vi "Acquire Data.vi"(7 "Total Buffer Size":i32 caption="全部缓冲区大小", 8 "error in (no error)":errorcluster caption="错误输入（无错误）", 10 "Acquisition and Logging Configuration":T2={"Samples per Read"=100, "Number of Reads to Save"=20, "Number of Channels"=4, "Channel Scale Array"=[1.0, 1.0, 1.0, 1.0], "Channel Names"=["Mod1\\AI0", "Mod1\\AI1", "Mod1\\AI2", "Mod1\\AI3"], "Trigger - RMS Value"=0.9999999999999994, "Trigger - Channel"=0, "Trigger - Time (Minute)"=10, "TDMS Properties"=[{"Name"="Company", "Value"="TongRui"}, {"Name"="Developer", "Value"="SUN"}], "Data File Name"="cRIO_Data", "Date Rate"=20} caption="采集与记录配置" {"Date Rate" items=["51.200 kS/s (NI 9234)"=1, "25.600 kS/s (NI 9234)"=2, "17.067 kS/s (NI 9234)"=3, "12.80 kS/s (NI 9234)"=4, "10.240 kS/s (NI 9234)"=5, "8.533 kS/s (NI 9234)"=6, "7.314 kS/s (NI 9234)"=7, "6.400 kS/s (NI 9234)"=8, "5.689 kS/s (NI 9234)"=9, "5.120 kS/s (NI 9234)"=10, "4.654 kS/s (NI 9234)"=11, "4.267 kS/s (NI 9234)"=12, "3.938 kS/s (NI 9234)"=13, "3.657 kS/s (NI 9234)"=14, "3.413 kS/s (NI 9234)"=15, "3.200 kS/s (NI 9234)"=16, "3.012 kS/s (NI 9234)"=17, "2.845 kS/s (NI 9234)"=18, "2.695 kS/s (NI 9234)"=19, "2.560 kS/s (NI 9234)"=20, "2.438 kS/s (NI 9234)"=21, "2.328 kS/s (NI 9234)"=22, "2.226 kS/s (NI 9234)"=23, "2.133 kS/s (NI 9234)"=24, "2.048 kS/s (NI 9234)"=25, "1.969 kS/s (NI 9234)"=26, "1.896 kS/s (NI 9234)"=27, "1.829 kS/s (NI 9234)"=28, "1.765 kS/s (NI 9234)"=29, "1.707 kS/s (NI 9234)"=30, "1.652 kS/s (NI 9234)"=31]}, 11 "FPGA VI Reference":T1 caption="FPGA VI引用") -> (0 "error out":errorcluster caption="错误输出", 1 "Waveform Data":waveform(sgl)[](array[waveform]) caption="波形数据", 2 "dup Acquisition and Logging Configuration":T2={"Samples per Read"=100, "Number of Reads to Save"=20, "Number of Channels"=4, "Channel Scale Array"=[1.0, 1.0, 1.0, 1.0], "Channel Names"=[], "Trigger - RMS Value"=0.9999999999999994, "Trigger - Channel"=0, "Trigger - Time (Minute)"=10, "TDMS Properties"=[], "Data File Name"="cRIO_Data", "Date Rate"=20} caption="采集与记录配置副本" {"Date Rate" items=["51.200 kS/s (NI 9234)"=1, "25.600 kS/s (NI 9234)"=2, "17.067 kS/s (NI 9234)"=3, "12.80 kS/s (NI 9234)"=4, "10.240 kS/s (NI 9234)"=5, "8.533 kS/s (NI 9234)"=6, "7.314 kS/s (NI 9234)"=7, "6.400 kS/s (NI 9234)"=8, "5.689 kS/s (NI 9234)"=9, "5.120 kS/s (NI 9234)"=10, "4.654 kS/s (NI 9234)"=11, "4.267 kS/s (NI 9234)"=12, "3.938 kS/s (NI 9234)"=13, "3.657 kS/s (NI 9234)"=14, "3.413 kS/s (NI 9234)"=15, "3.200 kS/s (NI 9234)"=16, "3.012 kS/s (NI 9234)"=17, "2.845 kS/s (NI 9234)"=18, "2.695 kS/s (NI 9234)"=19, "2.560 kS/s (NI 9234)"=20, "2.438 kS/s (NI 9234)"=21, "2.328 kS/s (NI 9234)"=22, "2.226 kS/s (NI 9234)"=23, "2.133 kS/s (NI 9234)"=24, "2.048 kS/s (NI 9234)"=25, "1.969 kS/s (NI 9234)"=26, "1.896 kS/s (NI 9234)"=27, "1.829 kS/s (NI 9234)"=28, "1.765 kS/s (NI 9234)"=29, "1.707 kS/s (NI 9234)"=30, "1.652 kS/s (NI 9234)"=31]})   [LabVIEW 2013]
doc: "读取DMA FIFO的波形数据。"
uses:
  controls/Acquisition and Logging Configuration.ctl
  controls/TDMS Properties.ctl
  <vilib>/LabVIEW Targets/FPGA/cRIO/shared/nicrio_ModuleControls/nicrio_cRIO-9234_DataRatesRing2.ctl
  controls/FPGA VI Reference.ctl
  <vilib>/rvi/interface/common/niFpgaWaitOnOcc.vi
  Globals/Global - Monitoring Variables.vi
  <vilib>/Utility/error.llb/Error Cluster From Error Code.vi
  <vilib>/rvi/errors/niLvFpgaAdjustHostInterfaceError.vi
  <vilib>/rvi/interface/nirviReadWriteControl/nirviReadWriteControl.xnode
  FPGA Bitfiles/LabVIEWFPGAWavef_FPGA_FPGAMain_vTbN89OLNVY.lvbitx
  FPGA Main.vi
  <vilib>/rvi/interface/nirviMethod/nirviMethod.xnode
  NiFpgaLv.dll
  <vilib>/FPGAPlugInAG/cRIO-9074/niLvFpga_ReadFifo_cRIO-9074.vi
  <vilib>/rvi/errors/niLvFpgaMergeErrorWithErrorCode.vi
panel:
  # "通道"
  # "保存"
  # "采样"
  # "触发"
  # "通道"
  # "保存"
  # "采样"
  # "触发"
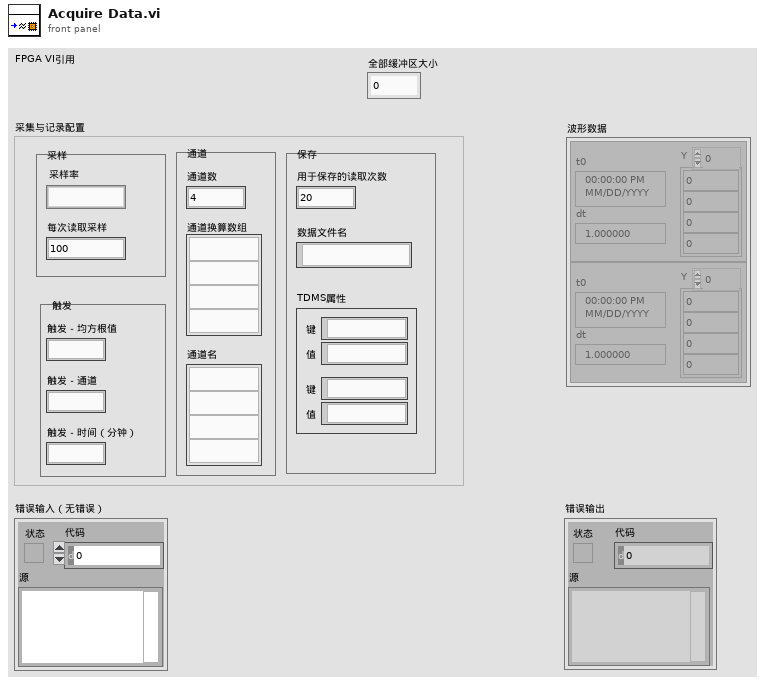
[diagram p1: front panel]
types:
  T1 = typedef "FPGA VI Reference.ctl" = refnum<k20>
  T2 = typedef "Acquisition and Logging Configuration.ctl" = cluster{"Samples per Read":i32, "Number of Reads to Save":i32, "Number of Channels":i32, "Channel Scale Array":fxp<+,24,12>[], "Channel Names":string[], "Trigger - RMS Value":dbl, "Trigger - Channel":i32, "Trigger - Time (Minute)":i32, "TDMS Properties":T3[], "Data File Name":string, "Date Rate":T4}
  T3 = typedef "TDMS Properties.ctl" = cluster{"Name":string, "Value":string}
  T4 = typedef "nicrio_cRIO-9234_DataRatesRing2.ctl" = u16
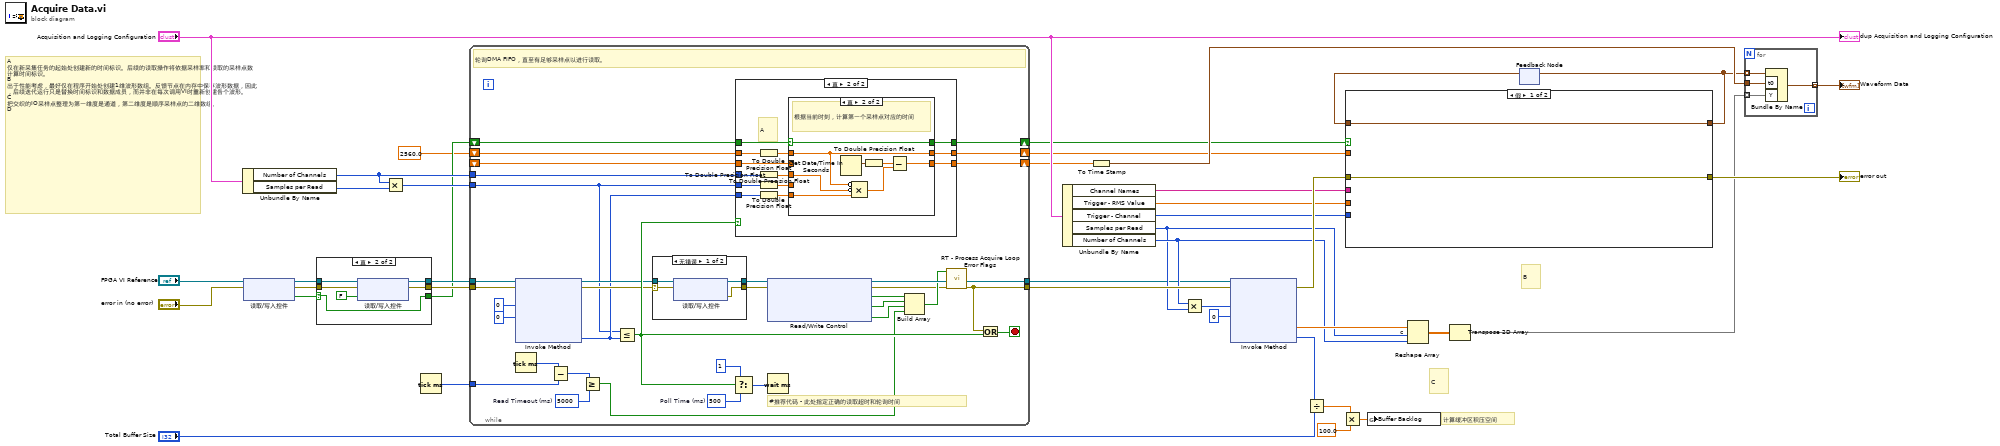
[diagram p0: block diagram]
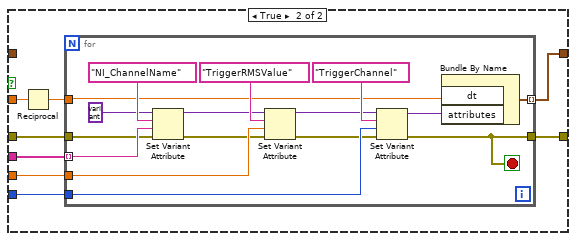
[diagram p2: hidden frame]
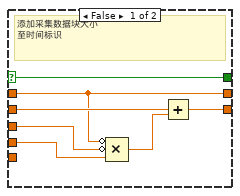
[diagram p5: hidden frame]
diagram:
  # "C"
  # "B"
  # "A\n仅在新采集任务的起始处创建新的时间标识。后续的读取操作将依据采样率和读取的采样点数计算时间标识。\nB\n出于性能考虑，最好仅在程序开始处创建1维波形数组。反馈节点在内存中保存波形数据，因此，后续迭代运行只是替换时间标识和数据成员，而并非在每次调用VI时重新创建各个波形。\nC\n把交织的IO采样点整理为第一维度是通道，第二维度是顺序采样点的二维数组。\nD"
  # "计算缓冲区积压空间"
  # "c"
  n1 = Unbundle By Name("Acquisition and Logging Configuration") -> ("Number of Channels"=w14:i32, "Samples per Read"=w15:i32)
  n2 = xnode "读取/写入控件"("FPGA VI引用输入"="FPGA VI Reference", "错误输入"="error in (no error)") -> ("FPGA VI引用输出"=w38:T1, "错误输出"=w39:errorcluster, "First Read"=w11:bool)
  n3 = case shown="真" w11 {
    selector: w11 -> [w41 w45]
    tunnel: w38 -> [w43 w49]
    tunnel: [w43 w48] -> w36
    tunnel: w39 -> [w42 w47]
    tunnel: [w42 w46] -> w35
    tunnel: [w41 w45] -> w10
    frame False {
    }
    frame True {
      n4 = xnode "读取/写入控件"("FPGA VI引用输入"=w49, "错误输入"=w47, "First Read"=FALSE) -> ("FPGA VI引用输出"=w48:T1, "错误输出"=w46:errorcluster)
    }
  }
  n5 = Multiply(x=w14, y=w15) -> (x*y=w30:i32)
  n6 = Tick Count (ms)() -> (millisecond timer value=w34:u32)
  n7 = while {
    tunnel: [w61] -> w33
    tunnel: [w66] -> w1
    tunnel: w36 -> [w81]
    tunnel: w35 -> [w80]
    shift-right: [w74] -> w32
    shift-left: _ -> [w79]
    tunnel: w34 -> [w82]
    tunnel: w30 -> [w50]
    tunnel: w14 -> [w58]
    shift-right: [w54] -> w13
    shift-left: 2560.0 -> [w59]
    shift-right: [w52] -> w12
    shift-left: w10 -> [w53]
    stop <- w83 stop-if-true
    w55 = u32 5000  # Read Timeout (ms)
    w56 = u32 500  # Poll Time (ms)
    # "#推荐代码 - 此处指定正确的读取超时和轮询时间"
    # "轮询DMA FIFO，直至有足够采样点以进行读取。"
    n8 = xnode "Invoke Method"("FPGA VI引用输入"=w81, "错误输入"=w80, "元素数量"=u32 0 ("Number of Elements"), "超时(ms)"=0 ("Timeout (ms)")) -> ("FPGA VI引用输出"=w69:T1, "错误输出"=w70:errorcluster, "剩余元素"=w51:u32)  [unwired: 1 out]
    n9 = Tick Count (ms)() -> (millisecond timer value=w78:u32)
    n10 = Subtract(x=w78, y=w82) -> (x-y=w71:u32)
    n11 = Greater Or Equal?(x=w71, y=w55) -> (x >= y?=w57:bool)
    n12 = Less Or Equal?(x=w50, y=w51) -> (x <= y?=w77:bool)
    n13 = case shown="无错误" w70 {
      selector: w70 -> [w87 w88]
      tunnel: w69 -> [w86 w89]
      tunnel: [w85 w89] -> w68
      tunnel: [w84 w88] -> w67
      frame No Error {
        n14 = xnode "读取/写入控件"("FPGA VI引用输入"=w86, "错误输入"=w87) -> ("FPGA VI引用输出"=w85:T1, "FPGA Error"=w84:errorcluster)  [unwired: 1 out]
      }
      frame Error {
      }
    }
    n15 = Select(t=u32 1, s=w77, f=w56) -> (s? t:f=w76:u32)
    n16 = case shown="真" w77 {
      tunnel: w79 -> [w92 w105]
      tunnel: w53 -> [w90 w104]
      tunnel: w51 -> [_ w103]
      tunnel: [w92 w102] -> w74
      tunnel: w50 -> [_ w101]
      tunnel: w59 -> [w91 w99]
      tunnel: w58 -> [_ w98]
      tunnel: [w91 w95] -> w54
      tunnel: [w90 w94] -> w52
      frame False {
      }
      frame True {
        # "A"
        n17 = To Double Precision Float(number=w99) -> (double precision float=w93:dbl)
        n18 = To Double Precision Float(number=w98) -> (double precision float=w100:dbl)
        n19 = To Double Precision Float(number=w101) -> (double precision float=w96:dbl)
        n20 = To Double Precision Float(number=w103) -> (double precision float=w97:dbl)
        n21 = case shown="真" w104 {
          selector: w104 -> [w106 w113]
          tunnel: w93 -> [w108 w115]
          tunnel: w105 -> [w111 _]
          tunnel: w96 -> [w109 _]
          tunnel: w100 -> [w110 w120]
          tunnel: w97 -> [_ w116]
          tunnel: [w112 w118] -> w102
          tunnel: [w108 w115] -> w95
          tunnel: [w106 w113] -> w94
          frame False {
            # "添加采集数据块大小\n至时间标识"
            n22 = Compound Arithmetic op=MULTIPLY(invert w108, invert w110, w109) -> (w107:dbl)
            n23 = Add(x=w111, y=w107) -> (x+y=w112:dbl)
          }
          frame True {
            # "根据当前时刻，计算第一个采样点对应的时间"
            n24 = Get Date/Time In Seconds() -> (seconds since 1Jan1904=w119:timestamp)
            n25 = Compound Arithmetic op=MULTIPLY(invert w115, invert w120, w116) -> (w114:dbl)
            n26 = To Double Precision Float(number=w119) -> (double precision float=w117:dbl)
            n27 = Subtract(x=w117, y=w114) -> (x-y=w118:dbl)
          }
        }
      }
    }
    n28 = xnode "Read/Write Control"("FPGA VI引用输入"=w68, "错误输入"=w67) -> ("FPGA VI引用输出"=w66:T1, "错误输出"=w60:errorcluster, "Module Underflow"=w63:bool, "DMA FIFO Full"=w65:bool, "Different Channel Count"=w64:bool)
    n29 = Wait (ms)(milliseconds to wait=w76) -> ()  [unwired: 1 out]
    n30 = Build Array(w63, w65, w64, w57) -> (w62:bool[])
    n31 = call "RT - Process Acquire Loop Error Flags.vi"("error in (no error)"=w60, "Error Flags"=w62) -> ("error out"=w61:errorcluster)  [unwired: 9 in]
    n32 = Or(x=w61, y=w77) -> (x .or. y?=w83:bool)
  }
  n33 = Unbundle By Name("Acquisition and Logging Configuration") -> ("Channel Names"=w4:string[], "Trigger - RMS Value"=w5:dbl, "Trigger - Channel"=w6:i32, "Samples per Read"=w7:i32, "Number of Channels"=w8:i32)
  n34 = To Time Stamp(1:w32) -> (0:w24:timestamp)
  n35 = Multiply(x=w8, y=w7) -> (x*y=w9:i32)
  n36 = xnode "Invoke Method"("FPGA VI引用输入"=w1, "错误输入"=w33, "元素数量"=w9, "超时(ms)"=0 ("Timeout (ms)")) -> ("错误输出"=w26:errorcluster, "数据"=w16:sgl[], "剩余元素"=w20:u32)  [unwired: 1 out]
  n37 = Divide(x=w20, y="Total Buffer Size") -> (x/y=w21:dbl)
  n38 = Multiply(x=w21, y=100.0) -> (x*y=w18:dbl)
  n39 = global write "Global - Monitoring Variables.vi" "Buffer Backlog"(w18) -> ()
  n40 = Reshape Array(w16, w7, w8) -> (w28:sgl[][])
  n41 = Transpose 2D Array(2D array=w28) -> (transposed array=w27:sgl[][])
  n42 = feedback #1 ("Initialized Waveforms")() -> (w22:waveform(sgl)[])  [unwired: 1 in]
  n43 = case shown="假" w12 {
    tunnel: w6 -> [_ w130]
    tunnel: w26 -> [w122 w129]
    tunnel: [w122 w128] -> w31
    tunnel: w5 -> [_ w127]
    tunnel: w4 -> [_ w126]
    tunnel: [w121 w125] -> w23
    tunnel: w22 -> [w121 _]
    tunnel: w13 -> [_ w124]
    frame False {
    }
    frame True {
      n44 = Reciprocal(x=w124) -> (1/x=w123:dbl)
      n45 = for {
        tunnel: w123 -> [w137]
        tunnel: [w146] -> w125 mode=indexing
        tunnel: w127 -> [w144]
        tunnel: w130 -> [w143]
        tunnel: w129 -> [w136]
        tunnel: [w138] -> w128
        tunnel: w126 -> [w139] mode=indexing
        stop <- w138 stop-if-true
        # "初始化波形属性"
        n46 = Set Variant Attribute(Variant=variant ("variant out"), name="NI_ChannelName", value=w139, error in=w136) -> (Variant out=w133:variant, error out=w134:errorcluster)  [unwired: 1 out]
        n47 = Set Variant Attribute(Variant=w133, name="TriggerRMSValue", value=w144, error in=w134) -> (Variant out=w131:variant, error out=w132:errorcluster)  [unwired: 1 out]
        n48 = Set Variant Attribute(Variant=w131, name="TriggerChannel", value=w143, error in=w132) -> (Variant out=w145:variant, error out=w138:errorcluster)  [unwired: 1 out]
        n49 = Bundle By Name("dt"=w137, "attributes"=w145) -> (w146:waveform(sgl))  [unwired: 1 out]
      }
    }
  }
  "error out" <- w31
  n50 = feedback-in #1(w23) -> ()
  n51 = for {
    tunnel: w23 -> [w150] mode=indexing
    tunnel: w24 -> [w149]
    tunnel: [w148] -> w29 mode=indexing
    tunnel: w27 -> [w147] mode=indexing
    n52 = Bundle By Name(cluster=w150, "t0"=w149, "Y"=w147) -> (w148:waveform(sgl))
  }
  "Waveform Data" <- w29
  "dup Acquisition and Logging Configuration" <- "Acquisition and Logging Configuration"
